vi "Configure Control Inhibit.vi"(7 "Unit Address (1)":u8=1, 8 "error in (no error)":errorcluster, 10 "Enable Control Inhibit (False)":bool, 11 "VISA resource name":refnum<visa-resource-name>) -> (0 "error out":errorcluster, 3 "VISA resource name out":refnum<visa-resource-name>)   [LabVIEW 2014, in "Eurotherm 35xx Series.lvlib"]
doc: "This VI is used to stop the loop controlling. If asserted the loop will stop control and the output of the loop will be set to the safe output value (SafeOutVal)."
uses:
  <instrlib>/Eurotherm 35xx Series/Eurotherm 35xx Series.lvlib
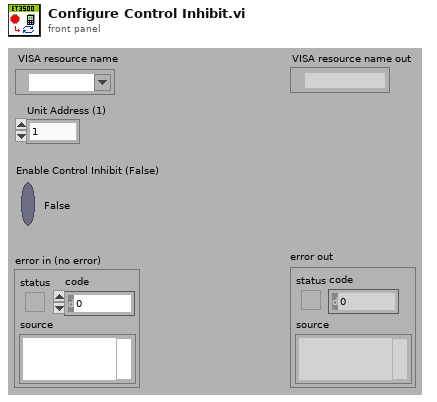
[diagram p1: front panel]
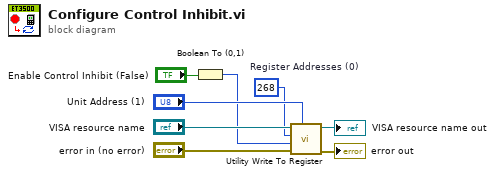
[diagram p0: block diagram]
diagram:
  w3 = 268  # Register Addresses (0)
  n1 = Boolean To (0,1)(Boolean="Enable Control Inhibit (False)") -> (0, 1=w1:i16)
  n2 = call <instrlib>:"Utility Write To Register.vi"("Unit Address (1)"="Unit Address (1)", "error in (no error)"="error in (no error)", "Data (0)"=w1, "Register Address (0)"=w3, "VISA resource name"="VISA resource name") -> ("error out"=→"error out":errorcluster, "VISA resource name out"=→"VISA resource name out":refnum<visa-resource-name>)  [unwired: 5 in]
